vi "to_json.vi"(8 "error in":errorcluster, 11 "datasflash in":refnum<class "datasflash.lvclass">) -> (0 "error out":errorcluster, 2 "json":string, 3 "datasflash out":refnum<class "datasflash.lvclass">, 4 "Not Default":bool)   [LabVIEW 2020, in "datasources.lvlib" / "datasflash.lvclass"]
uses:
  datasflash.lvclass
  C:/code/labview-client/lv_src/Nominal Client/datasources/datasource/datasource.lvclass
  datasource/datasource.lvclass/datasource.ctl
  4affb75b-fe6d-4066-acf3-3cd2b3337882.vi
  datasource/source.get.vi
  datasource/target.get.vi
  <vilib>/JDP Science/JSONtext/support/Format JSON Object.vi
  <vilib>/JDP Science/JSONtext/Variant to JSON Text.vi
  source/source.lvclass
  target/target.lvclass
  <vilib>/JDP Science/JSONtext/LVClass Serializer/JSONtext LVClass Serializer.lvclass
  datasflash.lvclass/datasflash.ctl
  <vilib>/JDP Science/JSONtext/JSONtext.lvlib
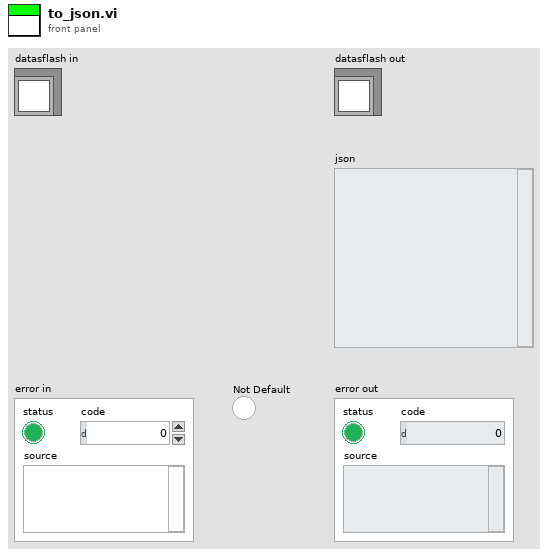
[diagram p1: front panel]
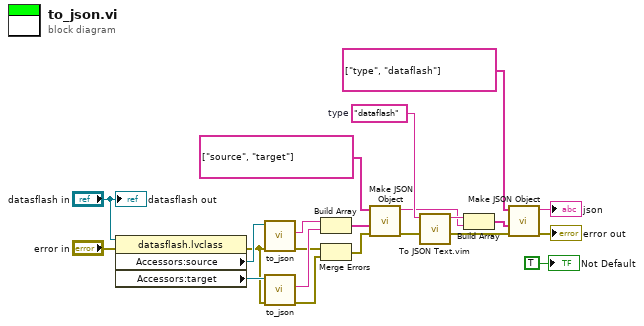
[diagram p0: block diagram]
diagram:
  w15 = "dataflash"  # type
  n1 = property class="datasflash.lvclass"(reference="datasflash in", error in="error in") -> (error out=w4:errorcluster, "Accessors:source"=w21:refnum<class "source.lvclass">, "Accessors:target"=w20:refnum<class "target.lvclass">)  [unwired: 1 out]
  n2 = call-dynamic "to_json.vi"("error in"=w4, "source in"=w21) -> ("error out"=w7:errorcluster, "json"=w19:string)  [unwired: 6 in, 2 out]
  n3 = call-dynamic "to_json.vi"("error in"=w4, "target in"=w20) -> ("error out"=w5:errorcluster, "json"=w18:string)  [unwired: 6 in, 2 out]
  n4 = Build Array(w19, w18) -> (w17:string[])
  n5 = Merge Errors(w7, w5) -> (w6:errorcluster)
  n6 = call <vilib>:"Make JSON Object.vi"("error in (no error)"=w6, "JSON Items"=w17, "Item Names"=string[] ["source", "target"]) -> ("error out"=w8:errorcluster, "<JSON>"=w13:string)  [unwired: 7 in]
  n7 = call "To JSON Text.vim"("error in (no error)"=w8, "Anything"=w15) -> ("error out"=w9:errorcluster, "<JSON>"=w14:string)  [unwired: 8 in]
  n8 = Build Array(w14, w13) -> (w12:string[])
  n9 = call <vilib>:"Make JSON Object.vi"("error in (no error)"=w9, "JSON Items"=w12, "Item Names"=string[] ["type", "dataflash"]) -> ("error out"=→"error out":errorcluster, "<JSON>"=→"json":string)  [unwired: 7 in]
  "datasflash out" <- "datasflash in"
  "Not Default" <- TRUE ("Not Default")
